vi "Database - Verify Existence.vi"(0 "reference in":refnum<class "Database_UUT.lvclass">, 5 "error in (no error)":errorcluster) -> (14 "reference out":refnum<class "Database_UUT.lvclass">, 18 "File Exists/Verified":bool, 19 "error out":errorcluster)   [LabVIEW 2017, in "Database_UUT.lvclass"]
uses:
  Database_UUT.lvclass
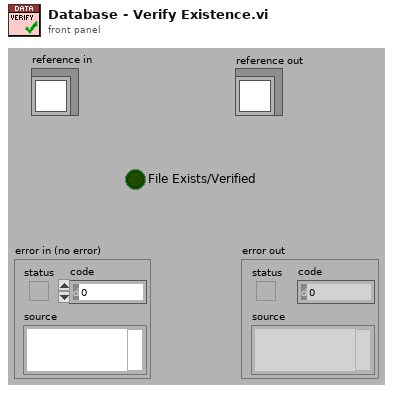
[diagram p1: front panel]
types:
  T1 = typedef "Database_UUT.lvclass/ObjectAttributes.ctl" = cluster{"Filepath to Database":path}
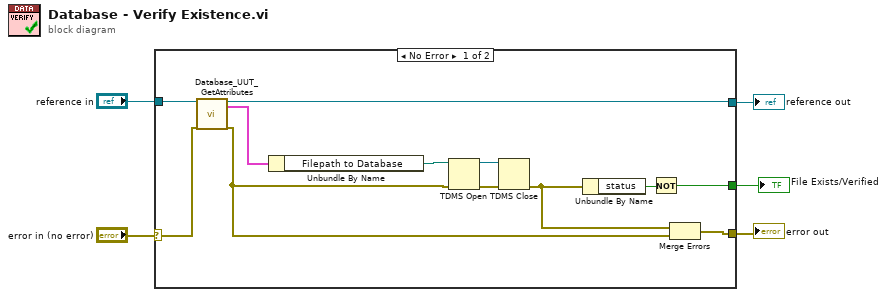
[diagram p0: block diagram]
diagram:
  n1 = case shown="No Error" "error in (no error)" {
    selector: "error in (no error)" -> [w16 w19]
    tunnel: [w14 w19] -> w4
    tunnel: [w15 w18] -> w2
    tunnel: "reference in" -> [w17 w18]
    tunnel: [w6 _] -> w1
    frame No Error {
      n2 = call "Database_UUT_GetAttributes.vi"("reference in"=w17, "error in (no error)"=w16) -> ("reference out"=w15:refnum<class "Database_UUT.lvclass">, "Data"=w13:T1, "error out"=w8:errorcluster)  [unwired: 14 in, 1 out]
      n3 = Unbundle By Name(w13) -> ("Filepath to Database"=w9:path)
      n4 = TDMS Open(8:w8, 11:w9) -> (0:w12:errorcluster, 3:w11:refnum<k34>)  [unwired: 5 in]
      n5 = TDMS Close(8:w12, 11:w11) -> (0:w7:errorcluster)  [unwired: 1 out]
      n6 = Unbundle By Name(w7) -> ("status"=w10:bool)
      n7 = Not(x=w10) -> (.not. x?=w6:bool)
      n8 = Merge Errors(w7, w8) -> (w14:errorcluster)
    }
    frame Error {
    }
  }
  "error out" <- w4
  "reference out" <- w2
  "File Exists/Verified" <- w1
